vi "PS FPGA Filter_Test.vi"(9 "filter?":bool, 11 "input":fxp<+/-,20,5>[](array[numeric])=[0.0, 0.0, 0.0, 0.0, 0.0, 0.0, 0.0, 0.0]) -> (2 "internal":fxp<+/-,20,5>[](array[numeric]), 3 "output":fxp<+/-,20,5>[](array[numeric]))   [LabVIEW 2011]
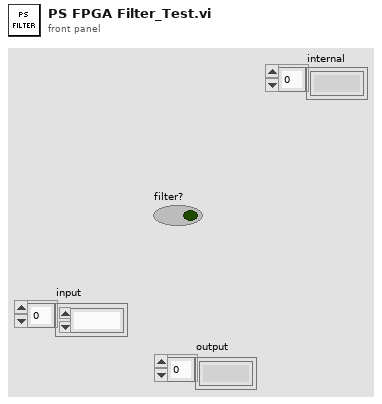
[diagram p1: front panel]
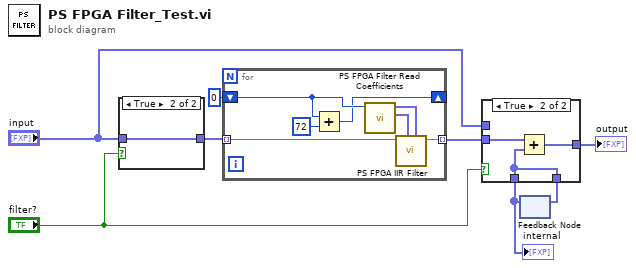
[diagram p0: block diagram]
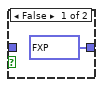
[diagram p2: hidden frame]
diagram:
  n1 = case shown="True" "filter?" {
    tunnel: "input" -> [_ w10]
    tunnel: [fxp<+/-,20,5>[] [0.0, 0.0, 0.0, 0.0, 0.0, 0.0, 0.0, 0.0] ("input") w10] -> w1
    frame False {
    }
    frame True {
    }
  }
  n2 = for {
    tunnel: w1 -> [w17] mode=indexing
    tunnel: [w16] -> w4 mode=indexing
    shift-right: [w12] -> _
    shift-left: u16 0 -> [w13]
    n3 = Add(x=w13, y=u16 72 ("Number of \nCoefficients\nper Channel")) -> (x+y=w12:u16)
    n4 = call "PS FPGA Filter Read Coefficients.vi"("offset"=w13) -> ("a coeffs"=w14:fxp<+/-,22,2>[], "b coeffs"=w15:fxp<+/-,22,2>[])  [unwired: 9 in]
    n5 = call "PS FPGA IIR Filter.vi"("coeff_b"=w15, "coeff_a"=w14, "input data"=w17) -> ("output data"=w16:fxp<+/-,20,5>)  [unwired: 8 in]
  }
  n6 = feedback #1() -> (w6:fxp<+/-,20,5>[])  [unwired: 1 in]
  "internal" <- w6
  n7 = case shown="True" "filter?" {
    tunnel: "input" -> [w18 _]
    tunnel: [w18 w21] -> w7
    tunnel: [w18 w19] -> w5
    tunnel: w6 -> [_ w19]
    tunnel: w4 -> [_ w20]
    frame False {
    }
    frame True {
      n8 = Add(x=w20, y=w19) -> (x+y=w21:fxp<+/-,20,5>[])
    }
  }
  "output" <- w7
  n9 = feedback-in #1(w5) -> ()
